vi "FTW-JSON-Escape.vi"(1 "String":string) -> (0 "Escaped UTF-8 String":string)   [LabVIEW 2013]
panel:
  # "Inputs"
  # "Outputs"
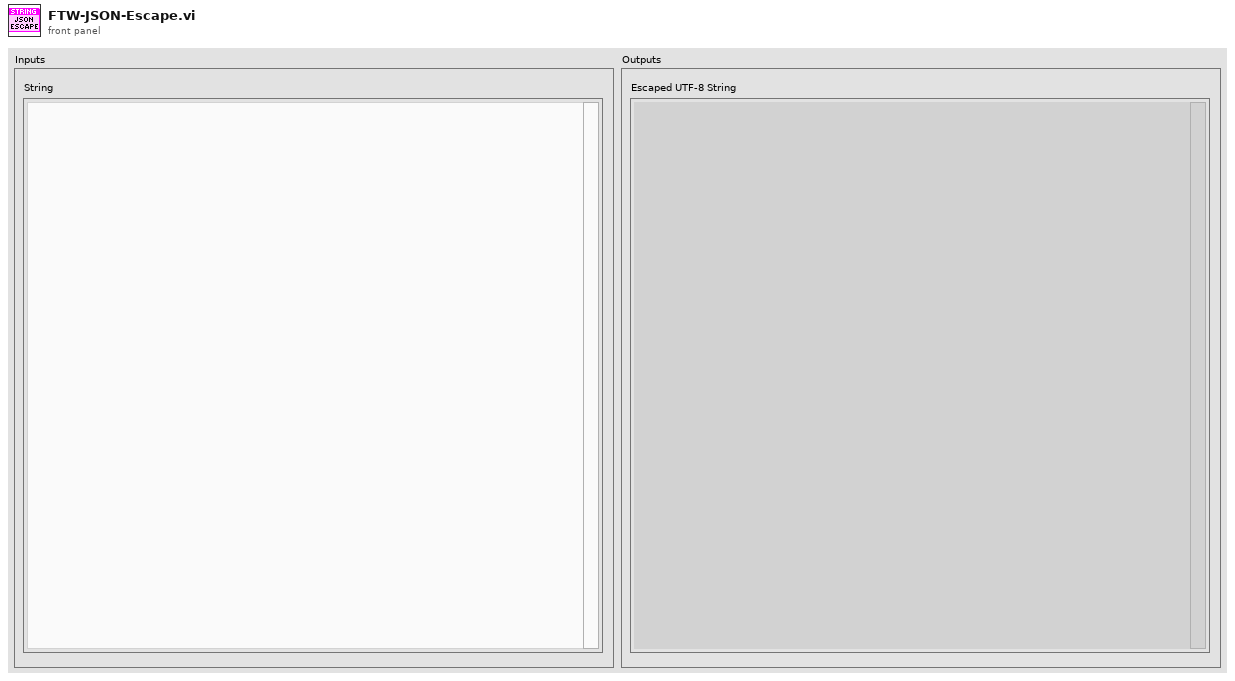
[diagram p1: front panel]
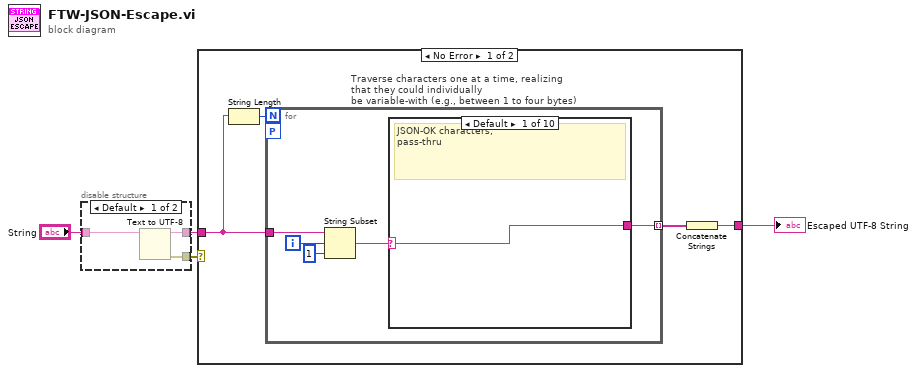
[diagram p0: block diagram]
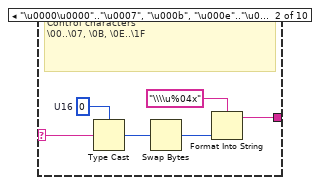
[diagram p3: hidden frame]
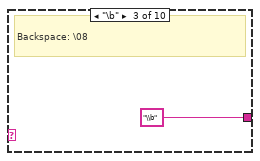
[diagram p4: hidden frame]
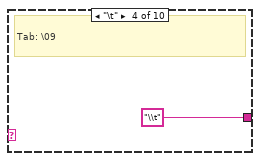
[diagram p5: hidden frame]
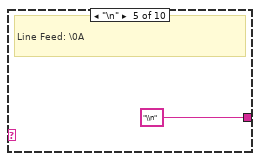
[diagram p6: hidden frame]
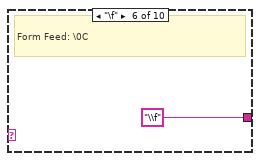
[diagram p7: hidden frame]
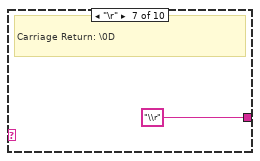
[diagram p8: hidden frame]
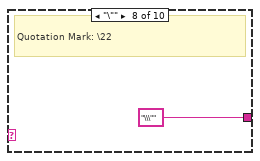
[diagram p9: hidden frame]
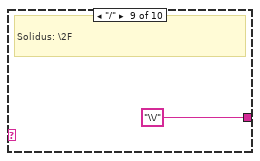
[diagram p10: hidden frame]
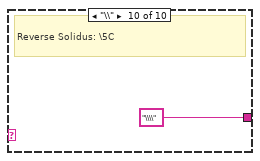
[diagram p11: hidden frame]
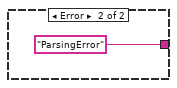
[diagram p12: hidden frame]
diagram:
  n1 = disable-structure shown="Default" {
    disable-tunnel: "String" -> [w7 w8]
    disable-tunnel: [w6 w8] -> w2
    disable-tunnel: [w5 _] -> w1
    frame condition #0 {
      n2 = Text to UTF-8(11:w7) -> (0:w5:errorcluster, 3:w6:string)  [unwired: 1 in]
    }
    frame condition #1 (active) {
    }
  }
  n3 = case shown="No Error" w1 {
    tunnel: [w11 "ParsingError" ("Escaped String")] -> w4
    tunnel: w2 -> [w10 _]
    frame No Error {
      n4 = String Length(string=w10) -> (length=w9:i32)
      n5 = for "Traverse characters one at a time, realizing that they could individually\nbe variable-with (e.g., between 1 to four bytes)" {
        N: w9 -> [_]
        tunnel: [w17] -> w12 mode=indexing
        tunnel: w10 -> [w16]
        workers-P: _ -> [_]
        i -> [w15]
        n6 = String Subset(string=w16, offset (0)=w15, length (rest)=1 ("length (rest)")) -> (substring=w13:string)
        n7 = case shown="Default" w13 {
          selector: w13 -> [w18 w22 _ _ _ _ _ _ _ _]
          tunnel: [w18 w23 "\\b" "\\t" "\\n" "\\f" "\\r" "\\\"" "\\/" "\\\\"] -> w17
          frame Default {
            # "JSON-OK characters;\npass-thru"
          }
          frame "\u0000\u0000".."\u0007", "\u000b", "\u000e".."\u001f" {
            w21 = u16 0  # U16
            # "Control characters\n\\00..\\07, \\0B, \\0E..\\1F"
            n8 = Type Cast(type=w21, x=w22) -> (*(type *) &x=w20:u16)
            n9 = Swap Bytes(anything=w20) -> (byte swapped=w19:u16)
            n10 = Format Into String(format string="\\\\u%04x", w19) -> (resulting string=w23:string)  [unwired: 2 in, 1 out]
          }
          frame "\b" {
            # "Backspace: \\08"
          }
          frame "\t" {
            # "Tab: \\09"
          }
          frame "\n" {
            # "Line Feed: \\0A"
          }
          frame "\f" {
            # "Form Feed: \\0C"
          }
          frame "\r" {
            # "Carriage Return: \\0D"
          }
          frame "\"" {
            # "Quotation Mark: \\22"
          }
          frame "/" {
            # "Solidus: \\2F"
          }
          frame "\\" {
            # "Reverse Solidus: \\5C"
          }
        }
      }
      n11 = Concatenate Strings(w12) -> (w11:string)
    }
    frame Error {
    }
  }
  "Escaped UTF-8 String" <- w4
